vi "GenerateCode.vi"(1 "Terms":T1[](array[typedef]), 3 "Diagram":refnum<vi>, 5 "XRef":refnum<vi>, 6 "State In":T4) -> (0 "Generated Code?":bool, 2 "State Out":T4, 4 "Reply":string[](array[string]))   [LabVIEW 2018, in "Foreign Key Sort.xnode"]
uses:
  Foreign Key Sort.xnode
  State.ctl
  <vilib>/XNodeSupport/XNodeTermIDPair.ctl
  <vilib>/XNodeSupport/XNodeTermRef.ctl
  <vilib>/XNodeSupport/XNodeString.ctl
  <vilib>/Utility/miscctls.llb/LVPositionTypeDef.ctl
  <userlib>/_LAVAcr/Scripting Tools/Scripting Tools.lvlib
  <vilib>/XNodeSupport/NI_XNodeSupport.lvlib
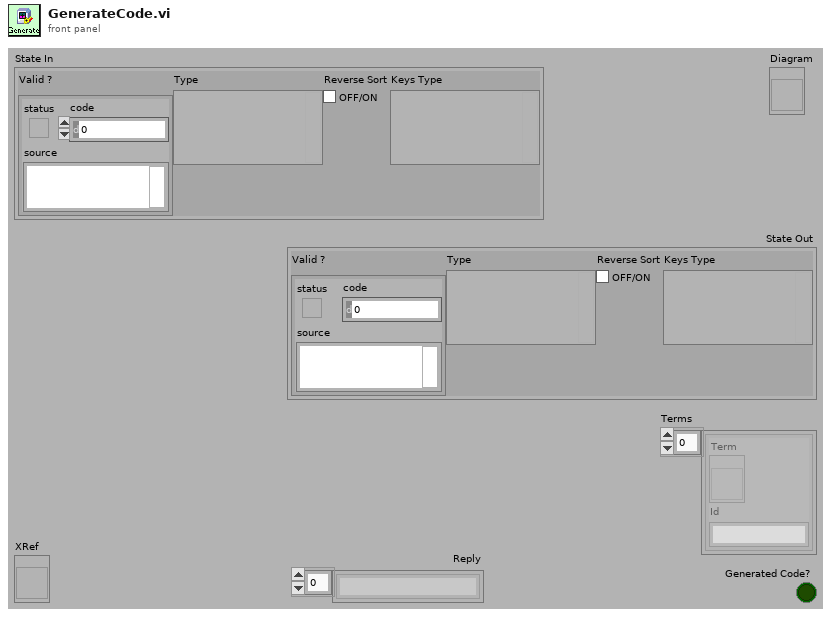
[diagram p1: front panel]
types:
  T1 = typedef "NI_XNodeSupport.lvlib/XNodeTermIDPair.ctl" = cluster{"Term":T2, "Id":T3}
  T2 = typedef "NI_XNodeSupport.lvlib/XNodeTermRef.ctl" = refnum<vi>
  T3 = typedef "NI_XNodeSupport.lvlib/XNodeString.ctl" = string
  T4 = typedef "Foreign Key Sort.xnode/State.ctl" = cluster{"Valid ?":errorcluster, "Type":variant, "Reverse Sort":bool, "Keys Type":variant}
  T5 = typedef "LVPositionTypeDef.ctl" = cluster{"Left":i32, "Top":i32}
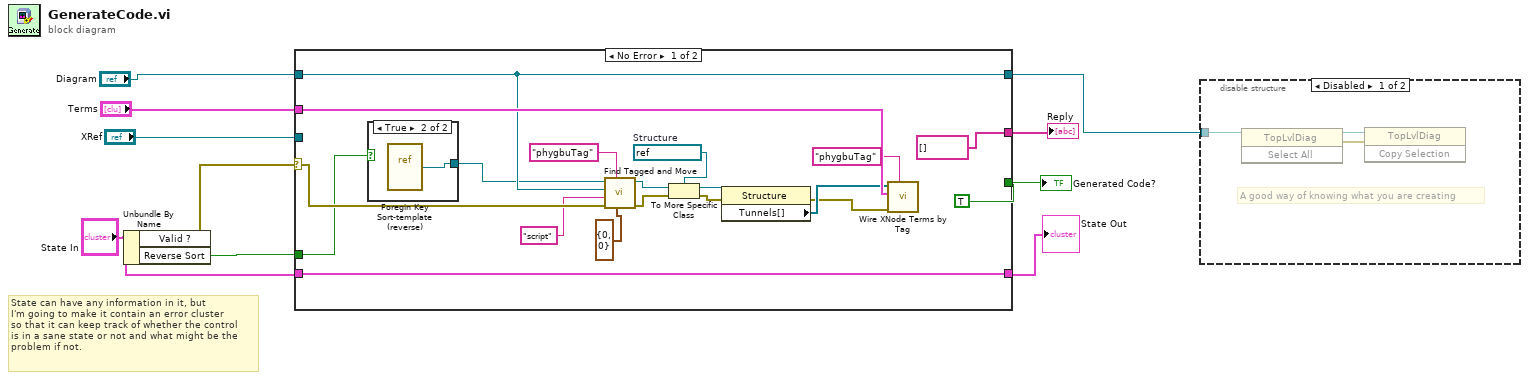
[diagram p0: block diagram]
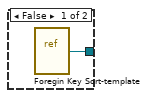
[diagram p2: hidden frame]
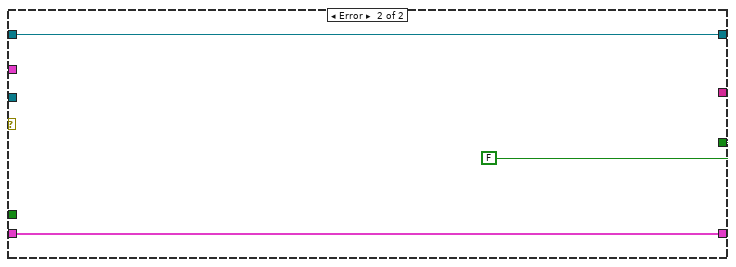
[diagram p3: hidden frame]
diagram:
  # "State can have any information in it, but\nI'm going to make it contain an error cluster\nso that it can keep track of whether the control\nis in a sane state or not and what might be the\nproblem if not."
  n1 = Unbundle By Name("State In") -> ("Valid ?"=w10:errorcluster, "Reverse Sort"=w1:bool)
  n2 = case shown="No Error" w10 {
    selector: w10 -> [w22 _]
    tunnel: "State In" -> [w27 w34]
    tunnel: "Diagram" -> [w21 w32]
    tunnel: "Terms" -> [w26 _]
    tunnel: "XRef" -> [_ _]
    tunnel: [w21 w32] -> w2
    tunnel: [string[] [] ("Reply") _] -> w5
    tunnel: [TRUE FALSE] -> w4
    tunnel: [w27 w34] -> w3
    tunnel: w1 -> [w11 _]
    frame No Error {
      w24 = refnum<vi> refnum  # Structure
      n3 = case shown="True" w11 {
        tunnel: [w30 w31] -> w12
        frame False {
          n4 = vi-ref "Foregin Key Sort-template.vi"() -> (w30:refnum<vi>)
        }
        frame True {
          n5 = vi-ref "Foregin Key Sort-template (reverse).vi"() -> (w31:refnum<vi>)
        }
      }
      n6 = call <userlib>:"Find Tagged and Move.vi"("position"=T5 {"Left"=0, "Top"=0}, "TagName"="phygbuTag", "error in"=w22, "TagValue"="script", "Destination Diagram"=w21, "VI Refnum"=w12) -> ("error out"=w16:errorcluster, "Moved Tagged object"=w17:refnum<vi>)  [unwired: 4 out]
      n7 = To More Specific Class(target class=w24, reference=w17, error in=w16) -> (specific class reference=w25:refnum<vi>, error out=w15:errorcluster)
      n8 = property class="Structure"(reference=w25, error in=w15) -> (error out=w14:errorcluster, "Tunnels[]"=w23:refnum<vi>[])  [unwired: 1 out]
      n9 = call <userlib>:"Wire XNode Terms by Tag.vi"("TagName"="phygbuTag", "error in (no error)"=w14, "Term Refs"=w26, "Source References"=w23) -> ()  [unwired: 8 out]
    }
    frame Error {
    }
  }
  "State Out" <- w3
  "Reply" <- w5
  "Generated Code?" <- w4
  n10 = disable-structure shown="Disabled" {
    disable-tunnel: w2 -> [w35 _]
    frame Disabled {
      # "A good way of knowing what you are creating"
      n11 = invoke class="TopLvlDiag" method="Select All"(reference=w35) -> (reference out=w37:refnum<vi>, error out=w36:errorcluster)  [unwired: 2 in, 1 out]
      n12 = invoke class="TopLvlDiag" method="Copy Selection"(reference=w37, error in=w36) -> ()  [unwired: 1 in, 3 out]
    }
    frame Enabled {
    }
  }
